vi "Read Reference.vi"(8 "error in (no error)":errorcluster, 11 "Chart in":refnum<class "Chart.lvclass">) -> (0 "error out":errorcluster, 2 "Reference":refnum<vi>, 3 "Chart out":refnum<class "Chart.lvclass">)   [LabVIEW 2019, in "Chart.lvclass"]
uses:
  Chart.lvclass
  Chart.lvclass/Chart.ctl
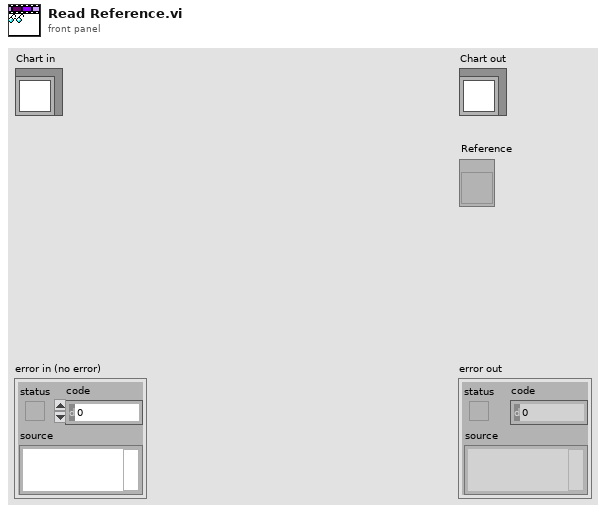
[diagram p1: front panel]
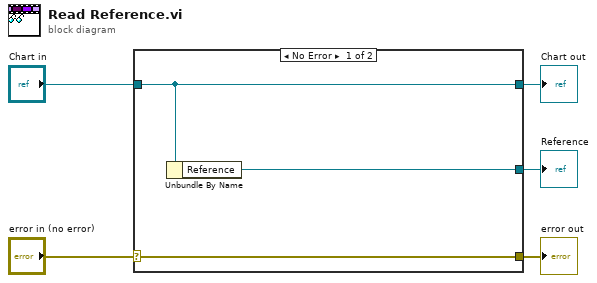
[diagram p0: block diagram]
diagram:
  n1 = case shown="No Error" "error in (no error)" {
    selector: "error in (no error)" -> [w8 w9]
    tunnel: [w8 w9] -> w4
    tunnel: [w7 w10] -> w2
    tunnel: "Chart in" -> [w7 w10]
    tunnel: [w6 _] -> w1
    frame No Error {
      n2 = Unbundle By Name(w7) -> ("Reference"=w6:refnum<vi>)
    }
    frame Error {
    }
  }
  "error out" <- w4
  "Chart out" <- w2
  "Reference" <- w1
